vi "GetControlValue.vi"(0 "reference in":refnum<class "MLA.lvclass">, 1 "Name":string, 5 "error in (no error)":errorcluster) -> (14 "reference out":refnum<class "MLA.lvclass">, 15 "Value":variant, 19 "error out":errorcluster)   [LabVIEW 2023, in "MLA.lvclass"]
uses:
  MLA.lvclass
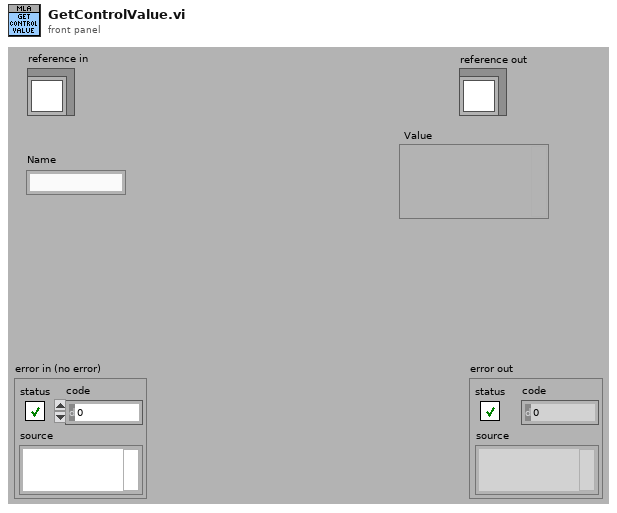
[diagram p1: front panel]
types:
  T1 = typedef "MLA.lvclass/ObjectAttributes.ctl" = cluster{"App Name":string, "App Version":string, "Revision History":string, "Log File Path":path, "Config INI File":path, "Config Path":path, "Log Archive Path":path, "Msg Q's":refnum<queue>[], "VI":refnum<vi>, "ErrLog":refnum<class "ErrorLog.lvclass">}
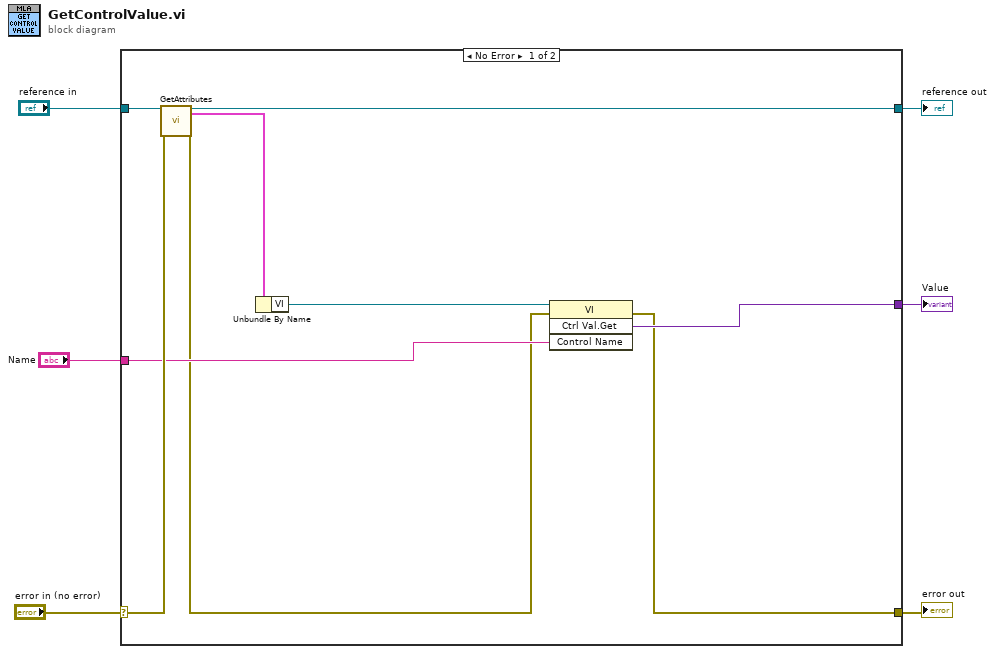
[diagram p0: block diagram]
diagram:
  n1 = case shown="No Error" "error in (no error)" {
    selector: "error in (no error)" -> [w15 w17]
    tunnel: [w7 w17] -> w5
    tunnel: [w12 w16] -> w3
    tunnel: "reference in" -> [w13 w16]
    tunnel: [w9 _] -> w2
    tunnel: "Name" -> [w10 _]
    frame No Error {
      n2 = call "GetAttributes.vi"("MLA"=w13, "error in (no error)"=w15) -> ("MLA"=w12:refnum<class "MLA.lvclass">, "Data"=w14:T1, "error out"=w8:errorcluster)  [unwired: 14 in, 1 out]
      n3 = Unbundle By Name(w14) -> ("VI"=w11:refnum<vi>)
      n4 = invoke class="VI" method="Ctrl Val.Get"(reference=w11, error in=w8, "Control Name"=w10) -> (error out=w7:errorcluster, "Get Control Value Variant"=w9:variant)  [unwired: 1 in, 2 out]
    }
    frame Error {
    }
  }
  "error out" <- w5
  "reference out" <- w3
  "Value" <- w2
